vi "VIWithTypeDefs.vi"(4 "Cluster":cluster{"Numeric":dbl, "String":string}, 5 "Invocation info":T2) -> (0 "error out":errorcluster, 2 "Test Data 2":T1 {"Numeric Measurement" format="%.2f"})   [LabVIEW 2012]
uses:
  <vilib>/addons/TestStand/_TSLegacy.llb/LabVIEW Test - Invocation Info.ctl
  <vilib>/addons/TestStand/_TSLegacy.llb/LabVIEW Test - Test Data.ctl
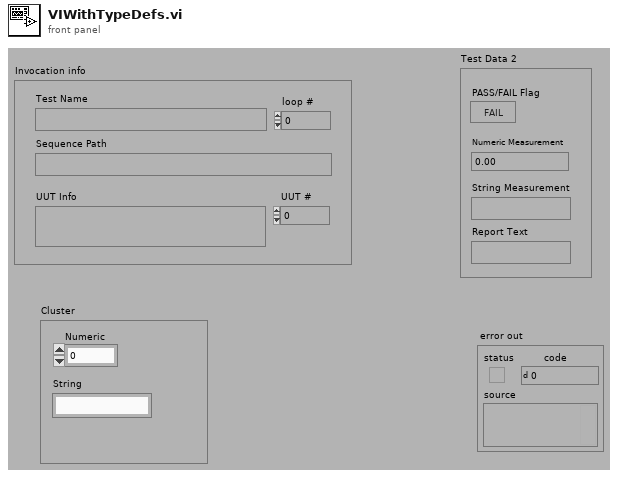
[diagram p1: front panel]
types:
  T1 = typedef "LabVIEW Test - Test Data.ctl" = cluster{"PASS/FAIL Flag":bool, "Numeric Measurement":dbl, "String Measurement":string, "Report Text":string}
  T2 = typedef "LabVIEW Test - Invocation Info.ctl" = cluster{"UUT #":i32, "loop #":i32, "UUT Info":string, "Test Name":string, "Sequence Path":path}
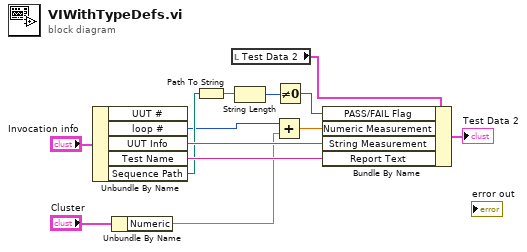
[diagram p0: block diagram]
diagram:
  n1 = Unbundle By Name("Invocation info") -> ("loop #"=w1:i32, "UUT Info"=w10:string, "Test Name"=w9:string, "Sequence Path"=w8:path)  [unwired: 1 out]
  n2 = Unbundle By Name("Cluster") -> ("Numeric"=w2:dbl)
  n3 = Path To String(path=w8) -> (string=w7:string)
  n4 = local read "Test Data 2"() -> (w12:T1)
  n5 = String Length(string=w7) -> (length=w5:i32)
  n6 = Add(x=w1, y=w2) -> (x+y=w4:dbl)
  n7 = Not Equal To 0?(x=w5) -> (x != 0?=w6:bool)
  n8 = Bundle By Name(cluster=w12, "PASS/FAIL Flag"=w6, "Numeric Measurement"=w4, "String Measurement"=w10, "Report Text"=w9) -> (→"Test Data 2":T1)
